vi "roboRIO v1.0 Build MUX Configuration PWM.vi"(11 "Channel":T4) -> (2 "Configuration Bitmask Array":bool[][](array[boolean]), 3 "Channel Reservation List":T1)   [LabVIEW 2021]
uses:
  <vilib>/myRIO/Common/Instrument Driver Framework/myRIO v1.0/PWM/typedefs/PWM Channels Enum.ctl
  <vilib>/myRIO/Common/Instrument Driver Framework/roboRIO v1.0/Resource Manager/typedefs/roboRIO v1.0 Channel Reservation List.ctl
  <vilib>/myRIO/Common/Instrument Driver Framework/roboRIO v1.0/Resource Manager/typedefs/roboRIO v1.0 Channel Reservation Info.ctl
  <vilib>/myRIO/Common/Instrument Driver Framework/roboRIO v1.0/Resource Manager/typedefs/roboRIO v1.0 Connector List.ctl
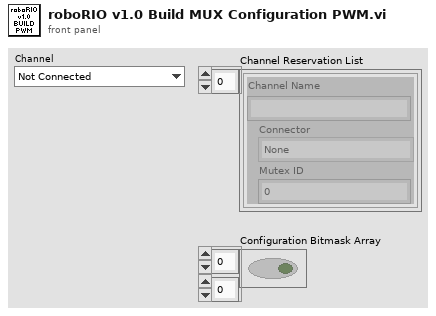
[diagram p1: front panel]
types:
  T1 = typedef "roboRIO v1.0 Channel Reservation List.ctl" = T2[]
  T2 = typedef "roboRIO v1.0 Channel Reservation Info.ctl" = cluster{"Channel Name":string, "Connector":T3, "Mutex ID":i32}
  T3 = typedef "roboRIO v1.0 Connector List.ctl" = enum32{"None", "ConnectorB", "ConnectorI2C", "ConnectorDIO", "ConnectorRSL", "ConnectorRELAY", "ConnectorAI", "ConnectorPWM", "ConnectorSPI"}
  T4 = typedef "PWM Channels Enum.ctl" = enum16{"Not Connected", "C/PWM0", "C/PWM1", "A/PWM0", "A/PWM1", "A/PWM2", "A/PWM3", "A/PWM4", "A/PWM5", "A/PWM6", "A/PWM7", "A/PWM8", "A/PWM9", "A/PWM10", "A/PWM11", "A/PWM12", "A/PWM13", "A/PWM14", "A/PWM15", "A/PWM16", "A/PWM17", "A/PWM18", "A/PWM19", "B/PWM0", "B/PWM1", "B/PWM2", "B/PWM3", "B/PWM4", "B/PWM5", "B/PWM6", "B/PWM7", "B/PWM8", "B/PWM9", "B/PWM10", "B/PWM11", "B/PWM12", "B/PWM13", "B/PWM14", "B/PWM15", "B/PWM16", "B/PWM17", "B/PWM18", "B/PWM19", "PWM/PWM0", "PWM/PWM1", "PWM/PWM2", "PWM/PWM3", "PWM/PWM4", "PWM/PWM5", "PWM/PWM6", "PWM/PWM7", "PWM/PWM8", "PWM/PWM9"}
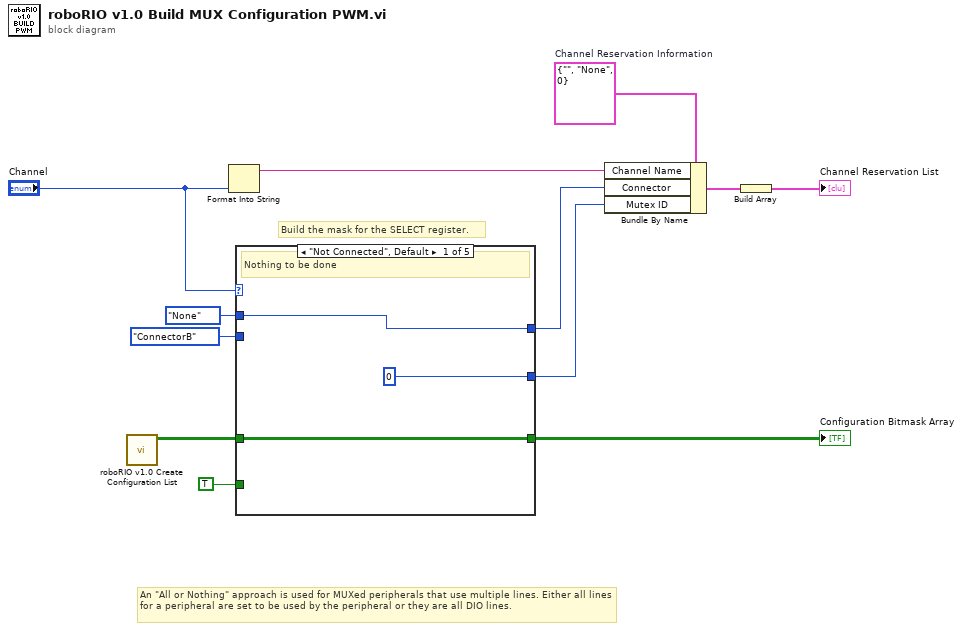
[diagram p0: block diagram]
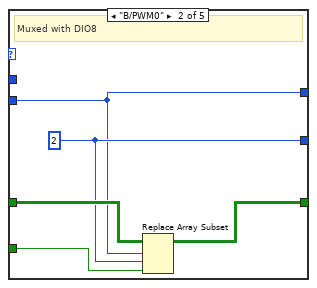
[diagram p2: hidden frame]
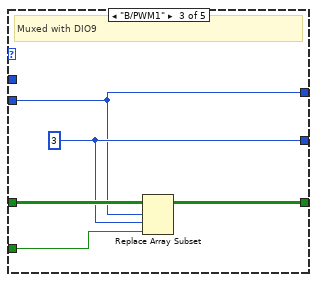
[diagram p3: hidden frame]
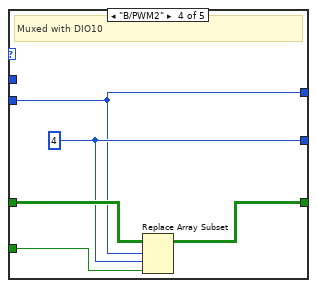
[diagram p4: hidden frame]
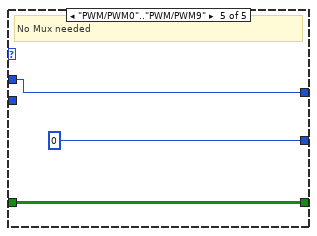
[diagram p5: hidden frame]
diagram:
  w7 = T2 {"Channel Name"="", "Connector"=enum."None", "Mutex ID"=0}  # Channel Reservation Information
  # "An \"All or Nothing\" approach is used for MUXed peripherals that use multiple lines. Either all lines for a peripheral are set to be used by the peripheral or they are all DIO lines."
  # "Build the mask for the SELECT register."
  n1 = call <vilib>:"roboRIO v1.0 Create Configuration List.vi"() -> ("Bitmask Array"=w8:bool[][])  [unwired: 11 in]
  n2 = Format Into String("Channel") -> (resulting string=w4:string)  [unwired: 3 in, 1 out]
  n3 = case shown="\"Not Connected\", Default" "Channel" {
    tunnel: w8 -> [w15 w20 w25 w30 w32]
    tunnel: [w15 w19 w24 w29 w32] -> w9
    tunnel: roboRIO_v1.0_Connector_List."None" ("Connector List") -> [w14 _ _ _ w31]
    tunnel: roboRIO_v1.0_Connector_List."ConnectorB" ("Connector List") -> [_ w16 w21 w26 _]
    tunnel: TRUE ("new element/subarray") -> [_ w18 w23 w28 _]
    tunnel: [0 ("index") w17 w22 w27 0 ("index")] -> w1
    tunnel: [w14 w16 w21 w26 w31] -> w2
    frame "Not Connected", Default {
      # "Nothing to be done"
    }
    frame "B/PWM0" {
      w17 = 2 ("index")
      # "Muxed with DIO8"
      n4 = Replace Array Subset(array=w20, new element=w18, index (row)=w16, index (col)=w17) -> (w19:bool[][])
    }
    frame "B/PWM1" {
      w22 = 3 ("index")
      # "Muxed with DIO9"
      n5 = Replace Array Subset(array=w25, new element=w23, index (row)=w21, index (col)=w22) -> (w24:bool[][])
    }
    frame "B/PWM2" {
      w27 = 4 ("index")
      # "Muxed with DIO10"
      n6 = Replace Array Subset(array=w30, new element=w28, index (row)=w26, index (col)=w27) -> (w29:bool[][])
    }
    frame "PWM/PWM0".."PWM/PWM9" {
      # "No Mux needed"
    }
  }
  "Configuration Bitmask Array" <- w9
  n7 = Bundle By Name(cluster=w7, "Channel Name"=w4, "Connector"=w2, "Mutex ID"=w1) -> (w6:T2)
  n8 = Build Array(w6) -> (→"Channel Reservation List":T2[])
